vi "ejemplo.vi"() -> ()   [LabVIEW 2020]
uses:
  <vilib>/ErrorRing/Error Ring.xnode
panel:
  in  "Nombre del Archivo":string
  in  "Formato":string(combo)
  in  "Direccion":path
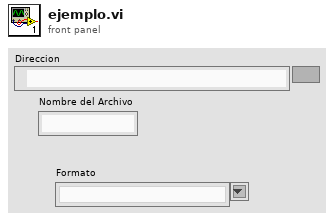
[diagram p1: front panel]
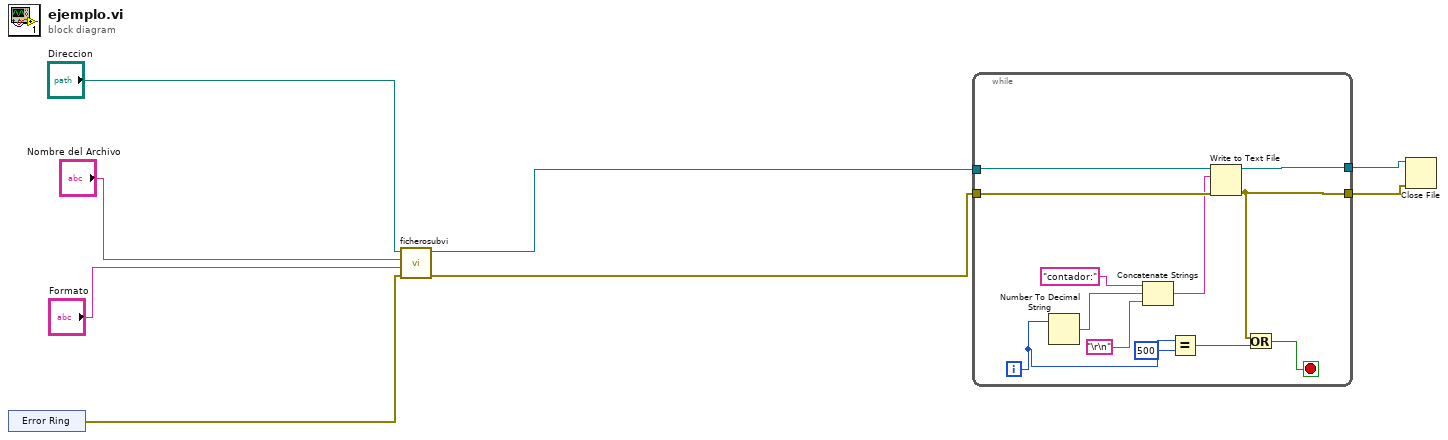
[diagram p0: block diagram]
diagram:
  n1 = xnode "Error Ring"() -> ("error out"=w5:errorcluster)
  n2 = call "ficherosubvi.vi"("error in (no error)"=w5, "Formato"="Formato", "Nombre del Archivo"="Nombre del Archivo", "Direccion"="Direccion") -> ("error out"=w3:errorcluster, "Byte Stream File out"=w4:refnum<file>)  [unwired: 6 in]
  n3 = while {
    tunnel: w4 -> [w20]
    tunnel: w3 -> [w19]
    tunnel: [w18] -> w2
    tunnel: [w14] -> w1
    i -> [w13]
    stop <- w10 stop-if-true
    n4 = Number To Decimal String(number=w13) -> (decimal integer string=w16:string)  [unwired: 1 in]
    n5 = Concatenate Strings("contador:", w16, "\r\n") -> (w9:string)
    n6 = Equal?(x=w13, y=500) -> (x = y?=w11:bool)
    n7 = Write to Text File(file (use dialog)=w20, text=w9, error in=w19) -> (refnum out=w18:refnum<file>, error out=w14:errorcluster)  [unwired: 1 in, 1 out]
    n8 = Or(x=w14, y=w11) -> (x .or. y?=w10:bool)
  }
  n9 = Close File(refnum=w2, error in=w1) -> ()  [unwired: 2 out]
